vi "hiwave.vi"(10 "等待时间（毫秒）":u32, 11 "路径":path) -> ()   [LabVIEW 2018]
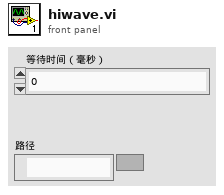
[diagram p1: front panel]
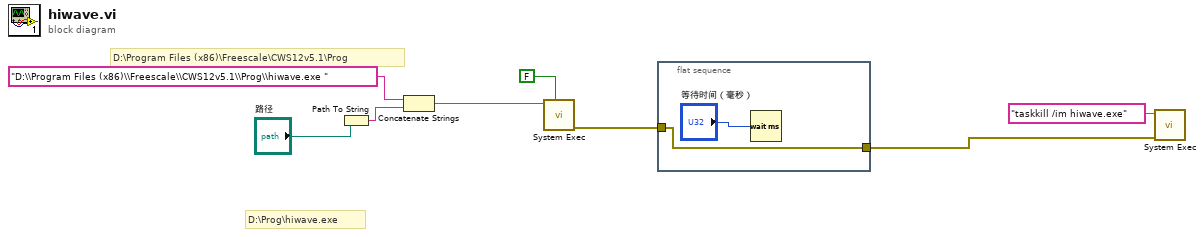
[diagram p0: block diagram]
diagram:
  # "D:\\Prog\\hiwave.exe"
  # "D:\\Program Files (x86)\\Freescale\\CWS12v5.1\\Prog"
  n1 = Path To String(path="路径") -> (string=w2:string)
  n2 = Concatenate Strings("D:\\Program Files (x86)\\Freescale\\CWS12v5.1\\Prog\\hiwave.exe " ("command line"), w2) -> (w3:string)
  n3 = call <vilib>:"System Exec.vi"("wait until completion? (T)"=FALSE, "command line"=w3) -> ("error out"=w8:errorcluster)  [unwired: 6 in, 3 out]
  n4 = flat-sequence {
    tunnel: w8 -> [w10]
    tunnel: [w10] -> w7
    frame #0 {
      n5 = Wait (ms)(milliseconds to wait="等待时间（毫秒）") -> ()  [unwired: 1 out]
    }
  }
  n6 = call <vilib>:"System Exec.vi"("error in (no error)"=w7, "command line"="taskkill /im hiwave.exe") -> ()  [unwired: 6 in, 4 out]
